vi "Handle Error.vi"(8 "error in (no error)":errorcluster, 11 "PVClient-Example in":refnum<class "PVClient-Example.lvclass">) -> (0 "error out":errorcluster, 2 "stop actor?":bool=TRUE, 3 "PVClient-Example out":refnum<class "PVClient-Example.lvclass">)   [LabVIEW 2014, in "PVClient-Example.lvlib" / "PVClient-Example.lvclass"]
doc: "(<B>Filename</B>: Actor Framework.lvlib:Actor.lvclass:Handle Error.vi)\n\nDefines how the actor handles an error that occurred while processing a message.\n\nBy default, this method does nothing except stop the actor. This method also treats error code 43 (coming from <B>error in</B>) as a sign that the actor shut down normally. In this situation, the Handle Error method does not return the error on <B>error out</B>, meaning the actor's caller will not receive it. All other error codes will be returned on <B>error out</B>.\n\nA descendant class may override this method to change this behavior."
uses:
  PVClient-Example.lvclass
  CSPP_Core/Actors/CS++BaseActor/CS++BaseActor.lvclass
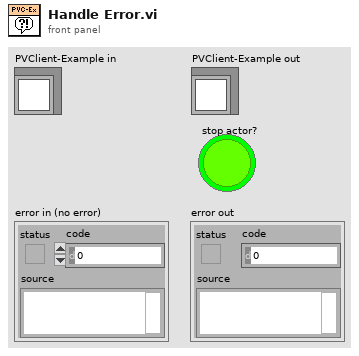
[diagram p1: front panel]
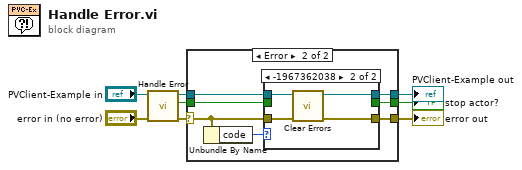
[diagram p0: block diagram]
diagram:
  n1 = call-parent "Handle Error.vi"("error in (no error)"="error in (no error)", "CS++BaseActor in"="PVClient-Example in") -> ("error out"=w6:errorcluster, "stop actor?"=w1:bool, "CS++BaseActor out"=w3:refnum<class "PVClient-Example.lvclass">)  [unwired: 7 in]
  n2 = case shown="Error" w6 {
    selector: w6 -> [w11 w16]
    tunnel: [w11 w17] -> w5
    tunnel: [w10 w14] -> w4
    tunnel: w3 -> [w10 w15]
    tunnel: [w9 w13] -> w2
    tunnel: w1 -> [w9 w12]
    frame No Error {
    }
    frame Error {
      n3 = Unbundle By Name(w16) -> ("code"=w18:i32)
      n4 = case shown="-1967362038" w18 {
        tunnel: [w21 w22] -> w17
        tunnel: w16 -> [w21 w24]
        tunnel: w15 -> [w20 w23]
        tunnel: [w20 w23] -> w14
        tunnel: [w19 _] -> w13
        tunnel: w12 -> [w19 _]
        frame Default {
        }
        frame -1967362038 {
          n5 = call <vilib>:"Clear Errors.vi"("error in (no error)"=w24) -> ("error out"=w22:errorcluster)  [unwired: 5 in, 1 out]
        }
      }
    }
  }
  "PVClient-Example out" <- w4
  "error out" <- w5
  "stop actor?" <- w2
